vi "Test2.vi"() -> ()   [LabVIEW 2021]
uses:
  <vilib>/myRIO/Instrument Drivers/Onboard IO/I2C/typedefs/I2C User Configuration.ctl
  <vilib>/myRIO/Instrument Drivers/Onboard IO/I2C/typedefs/I2C Transfer Rate.ctl
  <vilib>/myRIO/Instrument Drivers/Onboard IO/I2C/typedefs/I2C Reference.ctl
  <vilib>/myRIO/Common/Instrument Driver Framework/Utilities/typedefs/myRIO Generic Hardware Reference.ctl
  <vilib>/myRIO/Common/Instrument Driver Framework/Utilities/typedefs/Hardware Version Enum.ctl
  <vilib>/myRIO/Common/Instrument Driver Framework/Utilities/typedefs/myRIO v1.0 Reference.ctl
  <vilib>/myRIO/Common/Instrument Driver Framework/Utilities/typedefs/Generic FPGA Reference.ctl
  <vilib>/myRIO/Common/Instrument Driver Framework/myRIO v1.0/I2C/typedefs/I2C Channels Enum.ctl
  <vilib>/myRIO/Instrument Drivers/Onboard IO/I2C/typedefs/I2C Configuration.ctl
  <vilib>/userDefined/High Color/nirio_resource_hc.ctl
  <vilib>/myRIO/Common/Instrument Driver Framework/Utilities/vis/Is FPGA Ref Available.vi
  <vilib>/myRIO/Common/Instrument Driver Framework/myRIO v1.0/I2C/vis/myRIO v1.1 Open I2C.vi
  <vilib>/myRIO/Instrument Drivers/Onboard IO/I2C/vis/Configure.vi
  <vilib>/myRIO/Instrument Drivers/Onboard IO/I2C/vis/Write.vi
  <vilib>/myRIO/Instrument Drivers/Onboard IO/I2C/vis/Write Read.vi
  <vilib>/myRIO/Common/Instrument Driver Framework/Utilities/vis/Validate Channels.vi
  <vilib>/myRIO/Common/Instrument Driver Framework/myRIO v1.0/I2C/vis/myRIO v1.0 Reserve I2C.vi
  <vilib>/myRIO/Common/Instrument Driver Framework/myRIO v1.0/I2C/vis/myRIO v1.0 Build MUX Configuration I2C.vi
  <vilib>/myRIO/Common/Instrument Driver Framework/myRIO v1.0/Resource Manager/vis/myRIO v1.0 Reserve Channel List.vi
  <vilib>/myRIO/Common/Instrument Driver Framework/myRIO v1.0/Resource Manager/vis/myRIO v1.0 Create Configuration List.vi
  <vilib>/myRIO/Common/Instrument Driver Framework/myRIO v1.0/Resource Manager/vis/myRIO v1.0 Reserve Channel.vi
  <vilib>/myRIO/Common/Instrument Driver Framework/myRIO v1.0/Resource Manager/vis/myRIO v1.0 Unreserve Channel.vi
  <vilib>/myRIO/Common/Instrument Driver Framework/myRIO v1.0/Resource Manager/vis/myRIO v1.0 Build Mutex Name.vi
  <vilib>/Utility/VariantDataType/GetNumericInfo.vi
  <vilib>/Utility/error.llb/Error Cluster From Error Code.vi
  <vilib>/myRIO/Common/Instrument Driver Framework/myRIO v1.0/myRIO v1.1 Open.vi
  <vilib>/myRIO/Common/Instrument Driver Framework/Utilities/vis/IO Manager.vi
  <vilib>/myRIO/Common/Instrument Driver Framework/Utilities/vis/Configuration Manager.vi
  <vilib>/myRIO/Common/Instrument Driver Framework/myRIO v1.0/Resource Manager/vis/myRIO v1.0 Configure IO.vi
  <vilib>/myRIO/Common/Instrument Driver Framework/myRIO v1.0/myRIO v1.0 Close.vi
  <vilib>/myRIO/Common/Instrument Driver Framework/myRIO v1.0/I2C/vis/myRIO v1.0 Configure I2C.vi
  <vilib>/myRIO/Common/Instrument Driver Framework/myRIO v1.0/I2C/vis/myRIO v1.0 Write I2C.vi
  <vilib>/myRIO/Common/Instrument Driver Framework/myRIO v1.0/I2C/vis/myRIO v1.0 Read I2C.vi
  <vilib>/myRIO/Express VI/Onboard IO/I2C/I2C Express VI.xnode
  <vilib>/myRIO/Instrument Drivers/Onboard IO/I2C/vis/myRIO I2C Open.xnode
  <vilib>/myRIO/Instrument Drivers/Onboard IO/I2C/I2C.lvlib
panel:
  out "error out":errorcluster
  out "Bytes Read 5":u8[](array[numeric])
  out "Bytes Read 4":u8[](array[numeric])
  out "Boolean array 2":bool[](array[boolean])
  out "Who Am I":u8[](array[numeric])
  in  "error in (no error) 2":errorcluster
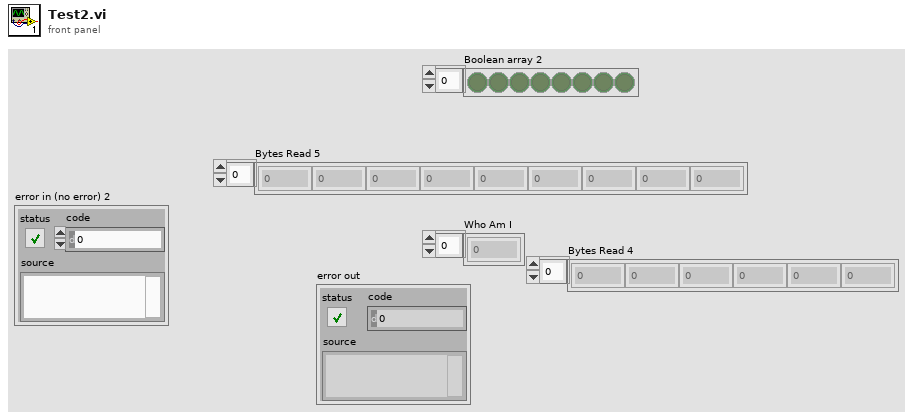
[diagram p1: front panel]
types:
  T1 = typedef "I2C.lvlib/I2C Reference.ctl" = cluster{"myRIO Reference":T2, "I2C Channels Enum":T6, "I2C Configuration":T7}
  T2 = typedef "myRIO Generic Hardware Reference.ctl" = cluster{"myRIO Model":T3, "myRIO Hardware Reference":T4}
  T3 = typedef "Hardware Version Enum.ctl" = enum16{"Unknown", "myRIO-1900", "myRIO-1950", "roboRIO", "NI ELVIS RIO CM", "ELVIS III"}
  T4 = typedef "myRIO v1.0 Reference.ctl" = cluster{"Generic FPGA Reference":T5, "Allow multiple opens":bool}
  T5 = typedef "Generic FPGA Reference.ctl" = refnum<k20>
  T6 = typedef "I2C Channels Enum.ctl" = enum16{"Not Connected", "A/I2C", "B/I2C", "I2C/I2C"}
  T7 = typedef "I2C.lvlib/I2C Configuration.ctl" = cluster{"I2C Transfer Rate":T8}
  T8 = typedef "I2C.lvlib/I2C Transfer Rate.ctl" = enum16{"Standard mode (100 kbps)", "Fast mode (400 kbps)"}
  T9 = typedef "I2C.lvlib/I2C User Configuration.ctl" = cluster{"I2C Transfer Rate":T8}
  T10 = typedef "nirio_resource_hc.ctl" = tag
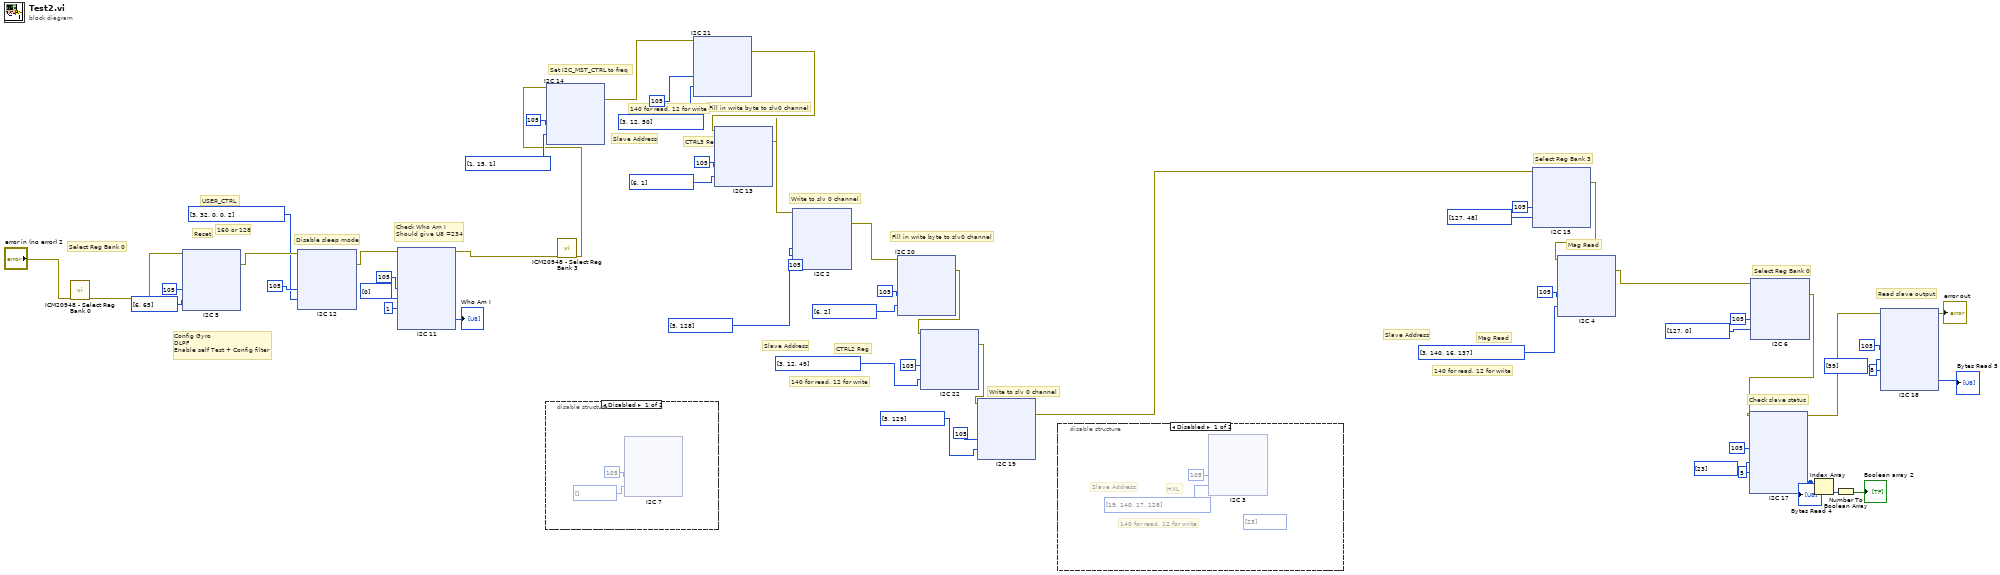
[diagram p0: block diagram]
diagram:
  # "CTRL2 Reg"
  # "Slave Address"
  # "140 for read, 12 for write"
  # "140 for read, 12 for write"
  # "CTRL3 Reg"
  # "Slave Address"
  # "USER_CTRL"
  # "Write to slv 0 channel"
  # "Fill in write byte to slv0 channel"
  # "Mag Read"
  # "Read slave output"
  # "Check slave status"
  # "Write to slv 0 channel"
  # "Fill in write byte to slv0 channel"
  # "160 or 128"
  # "Select Reg Bank 0"
  # "Set I2C_MST_CTRL to freq"
  # "Select Reg Bank 3"
  # "Check Who Am I \nShould give U8 =234"
  # "Disable sleep mode"
  # "Config Gyro\nDLPF\nEnable self Test + Config filter"
  # "Reset"
  # "Select Reg Bank 0"
  # "Mag Read"
  # "Slave Address"
  # "140 for read, 12 for write"
  n1 = call "ICM20948 - Select Reg Bank 0.vi"("error in (no error)"="error in (no error) 2") -> ("error out"=w45:errorcluster)  [unwired: 10 in]
  n2 = xnode "I2C 5"("Slave Address (7-bit)"=u8 105, "Bytes to Write"=u8[] [6, 65], "error in (no error)"=w45) -> ("error out"=w52:errorcluster)
  n3 = xnode "I2C 12"("Slave Address (7-bit)"=u8 105, "Bytes to Write"=u8[] [3, 32, 0, 0, 2], "error in (no error)"=w52) -> ("error out"=w41:errorcluster)
  n4 = xnode "I2C 11"("Slave Address (7-bit)"=u8 105, "Bytes to Write"=u8[] [0], "Byte Count"=u32 1, "error in (no error)"=w41) -> ("Bytes Read"=→"Who Am I":u8[], "error out"=w1:errorcluster)
  n5 = disable-structure shown="Disabled" {
    frame Disabled {
      n6 = xnode "I2C 7"("Slave Address (7-bit)"=u8 105, "Bytes to Write"=u8[] []) -> ()  [unwired: 1 in, 1 out]
    }
    frame Enabled {
    }
  }
  n7 = call "ICM20948 - Select Reg Bank 3.vi"("error in (no error)"=w1) -> ("error out"=w32:errorcluster)  [unwired: 10 in]
  n8 = xnode "I2C 14"("Slave Address (7-bit)"=u8 105, "Bytes to Write"=u8[] [1, 15, 1], "error in (no error)"=w32) -> ("error out"=w9:errorcluster)
  n9 = xnode "I2C 21"("Slave Address (7-bit)"=u8 105, "Bytes to Write"=u8[] [3, 12, 50], "error in (no error)"=w9) -> ("error out"=w8:errorcluster)
  n10 = xnode "I2C 13"("Slave Address (7-bit)"=u8 105, "Bytes to Write"=u8[] [6, 1], "error in (no error)"=w8) -> ("error out"=w35:errorcluster)
  n11 = xnode "I2C 2"("Slave Address (7-bit)"=u8 105, "Bytes to Write"=u8[] [5, 128], "error in (no error)"=w35) -> ("error out"=w12:errorcluster)
  n12 = xnode "I2C 20"("Slave Address (7-bit)"=u8 105, "Bytes to Write"=u8[] [6, 2], "error in (no error)"=w12) -> ("error out"=w4:errorcluster)
  n13 = xnode "I2C 22"("Slave Address (7-bit)"=u8 105, "Bytes to Write"=u8[] [3, 12, 49], "error in (no error)"=w4) -> ("error out"=w3:errorcluster)
  n14 = xnode "I2C 19"("Slave Address (7-bit)"=u8 105, "Bytes to Write"=u8[] [5, 129], "error in (no error)"=w3) -> ("error out"=w2:errorcluster)
  n15 = disable-structure shown="Disabled" {
    frame Disabled {
      (unwired) u8[] [23]
      # "HXL"
      # "Slave Address"
      # "140 for read, 12 for write"
      n16 = xnode "I2C 3"("Slave Address (7-bit)"=u8 105, "Bytes to Write"=u8[] [19, 140, 17, 128]) -> ()  [unwired: 1 in, 1 out]
    }
    frame Enabled {
    }
  }
  n17 = xnode "I2C 15"("Slave Address (7-bit)"=u8 105, "Bytes to Write"=u8[] [127, 48], "error in (no error)"=w2) -> ("error out"=w36:errorcluster)
  n18 = xnode "I2C 4"("Slave Address (7-bit)"=u8 105, "Bytes to Write"=u8[] [3, 140, 16, 137], "error in (no error)"=w36) -> ("error out"=w18:errorcluster)
  n19 = xnode "I2C 6"("Slave Address (7-bit)"=u8 105, "Bytes to Write"=u8[] [127, 0], "error in (no error)"=w18) -> ("error out"=w17:errorcluster)
  n20 = xnode "I2C 17"("Slave Address (7-bit)"=u8 105, "Bytes to Write"=u8[] [23], "Byte Count"=u32 5, "error in (no error)"=w17) -> ("Bytes Read"=w26:u8[], "error out"=w19:errorcluster)
  "Bytes Read 4" <- w26
  n21 = Index Array(array=w26) -> (element=w25:u8)  [unwired: 1 in]
  n22 = Number To Boolean Array(number=w25) -> (Boolean array=→"Boolean array 2":bool[])
  n23 = xnode "I2C 18"("Slave Address (7-bit)"=u8 105, "Bytes to Write"=u8[] [59], "Byte Count"=u32 8, "error in (no error)"=w19) -> ("Bytes Read"=→"Bytes Read 5":u8[], "error out"=→"error out":errorcluster)
